vi "GFITS_LibInitExtensions.vi"(8 "error in (no error)":errorcluster) -> (0 "error out":errorcluster, 2 "return value":i32)   [LabVIEW 2016]
uses:
  c/lib/libgfits.so
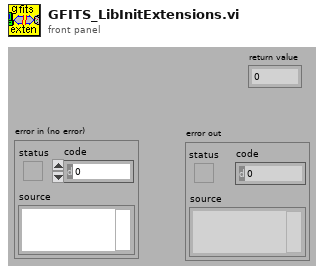
[diagram p1: front panel]
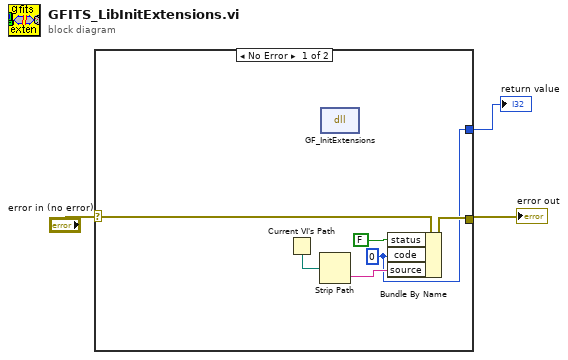
[diagram p0: block diagram]
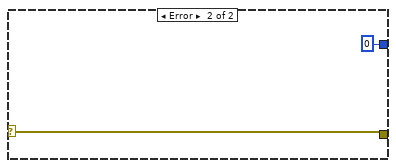
[diagram p2: hidden frame]
diagram:
  n1 = case shown="No Error" "error in (no error)" {
    selector: "error in (no error)" -> [w9 w11]
    tunnel: [w4 0] -> w3
    tunnel: [w6 w11] -> w1
    frame No Error {
      w4 = 0 ("code")
      n2 = Current VI's Path() -> (path=w8:path)
      n3 = Strip Path(path=w8) -> (name=w7:string)  [unwired: 1 out]
      n4 = dll-call lib="home/simager/panview/PAN/Modules/GFITS/private/c/lib/libgfits.so" fn="GF_InitExtensions"() -> ()  [unwired: 3 in, 3 out]
      n5 = Bundle By Name(cluster=w9, "status"=FALSE, "code"=w4, "source"=w7) -> (w6:errorcluster)
    }
    frame Error {
    }
  }
  "return value" <- w3
  "error out" <- w1
